vi "PH_Switch.PC Write PSDB.vi"(0 "i ref in":refnum<vi>, 5 "error IO":errorcluster) -> (14 "i ref out":refnum<vi>, 19 "error out":errorcluster)   [LabVIEW 2014, in "PH_Switch.lvlib"]
doc: "This is the proc case which writes data to the PHELIX shot data base."
uses:
  PH_Switch.lvlib
  PH_Basics/PH_PSDBWriter/PH_PSDBWriter.lvlib
  PH_Basics/PH_StatusHandler/PH_StatusHandler.lvlib
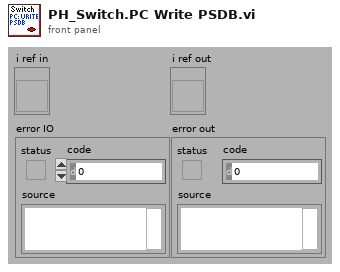
[diagram p1: front panel]
types:
  T1 = typedef "PH_Switch.lvlib/PH_Switch.i attribute.ctl" = cluster{"GUI Refs":T2, "Status true":T3, "Status false":T3, "Status Switch State":T3, "remote controlled":bool, "Tagname":cluster{"Switch":string, "True":string, "False":string}, "Beckhoff Instance":string, "Caption":cluster{"True":string, "False":string}, "Default State":string}
  T2 = typedef "PH_Switch.lvlib/PH_Switch.GUI Refs.ctl" = cluster{"true":refnum<vi>, "false":refnum<vi>, "Switch_state":refnum<vi>, "GUI-Knob":refnum<vi>, "Delete":refnum<vi>, "Function Textfield":refnum<vi>}
  T3 = typedef "PH_StatusHandler.lvlib/PH_StatusHandler.Status.ctl" = i16
  T4 = typedef "PH_PSDBWriter.lvlib/PH_PSDBWriter.String dataset.ctl" = cluster{"name":string, "data":string, "unit":string}
  T5 = typedef "PH_PSDBWriter.lvlib/PH_PSDBWriter.PSDB Dataset.ctl" = cluster{"Version":i32, "2D data Input":T6[], "Boolean Input":T8[], "Image Input":T9[], "Numeric Input":T11[], "String Input":T4[]}
  T6 = typedef "PH_PSDBWriter.lvlib/PH_PSDBWriter.2D dataset.ctl" = cluster{"name":string, "data":dbl[][], "axis description":T7}
  T7 = typedef "PSDB.lvlib/PSDB_AxisDescription.ctl" = cluster{"x axis label":string, "y axis label":string, "x axis unit":string, "y axis unit":string}
  T8 = typedef "PH_PSDBWriter.lvlib/PH_PSDBWriter.Boolean dataset.ctl" = cluster{"name":string, "data":bool, "unit":string}
  T9 = typedef "PH_PSDBWriter.lvlib/PH_PSDBWriter.Image dataset.ctl" = cluster{"name":string, "data":T10, "unit":string}
  T10 = typedef "IMAQ Image.ctl" = refnum<image>
  T11 = typedef "PH_PSDBWriter.lvlib/PH_PSDBWriter.Numeric dataset.ctl" = cluster{"name":string, "data":dbl, "unit":string}
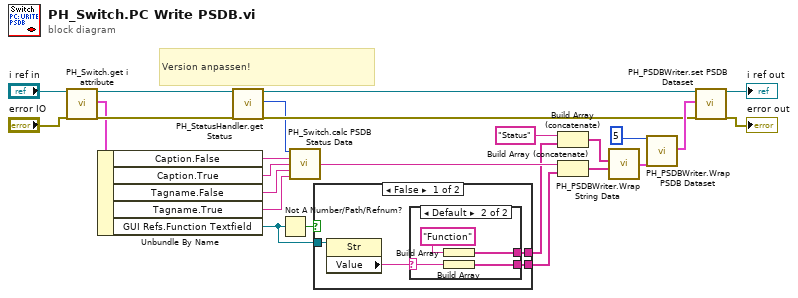
[diagram p0: block diagram]
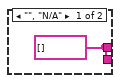
[diagram p2: hidden frame]
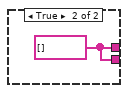
[diagram p3: hidden frame]
diagram:
  # "Version anpassen!"
  n1 = call "PH_Switch.get i attribute.vi"("i ref in"="i ref in", "error in (no error)"="error IO") -> ("i ref out"=w3:refnum<vi>, "i attribute"=w24:T1, "error out"=w25:errorcluster)  [unwired: 15 in]
  n2 = Unbundle By Name(w24) -> ("Caption.False"=w12:string, "Caption.True"=w11:string, "Tagname.False"=w10:string, "Tagname.True"=w9:string, "GUI Refs.Function Textfield"=w8:refnum<vi>)
  n3 = call "PH_StatusHandler.get Status.vi"("VI in"=w3, "error in"=w25) -> ("VI out"=w2:refnum<vi>, "Status"=w1:T3, "error out"=w4:errorcluster)  [unwired: 15 in]
  n4 = Not A Number/Path/Refnum?(number/path/refnum=w8) -> (NaN/Path/Refnum?=w7:bool)
  n5 = call "PH_Switch.calc PSDB Status Data.vi"("Status"=w1, "caption false"=w12, "caption true"=w11, "Tagname false"=w10, "Tagname true"=w9) -> ("PSDB Status"=w18:string)  [unwired: 10 in]
  n6 = case shown="False" w7 {
    tunnel: w8 -> [w28 _]
    tunnel: [w27 w35] -> w6
    tunnel: [w26 w35] -> w5
    frame False {
      n7 = property class="Str"(reference=w28) -> ("Value"=w29:string)  [unwired: 1 in, 2 out]
      n8 = case shown="Default" w29 {
        selector: w29 -> [_ w34]
        tunnel: [w30 w32] -> w26
        tunnel: [w30 w31] -> w27
        frame "", "N/A" {
          w30 = string[] []
        }
        frame Default {
          n9 = Build Array("Function" ("Caption In")) -> (w31:string[])
          n10 = Build Array(w34) -> (w32:string[])
        }
      }
    }
    frame True {
      w35 = string[] []
    }
  }
  n11 = Build Array (concatenate)("Status" ("name"), w6) -> (w16:string[])
  n12 = Build Array (concatenate)(w18, w5) -> (w15:string[])
  n13 = call "PH_PSDBWriter.Wrap String Data.vi"("Data Array"=w15, "Name Array"=w16) -> ("PSDB String Data Array"=w19:T4[])  [unwired: 2 in]
  n14 = call "PH_PSDBWriter.Wrap PSDB Dataset.vi"("Version"=5, "String Input"=w19) -> ("PSDB Dataset"=w20:T5)  [unwired: 17 in]
  n15 = call "PH_PSDBWriter.set PSDB Dataset.vi"("VI in"=w2, "PSDB Dataset"=w20, "error in (no error)"=w4) -> ("VI out"=→"i ref out":refnum<vi>, "error out"=→"error out":errorcluster)  [unwired: 15 in]
